vi "GetSetCtrls.vi"(8 "error in (no error)":errorcluster, 10 "Function (Load)":enum16{"Load", "Save"}(ring), 11 "Ini file (empty)":path) -> (0 "error out":errorcluster)   [LabVIEW 2011]
panel:
  out "Saved data":cluster{"Name":string, "Variant Data":variant}[](array[cluster])
  out "Initialized data":cluster{"Name":string, "Variant Data":variant}[](array[cluster])
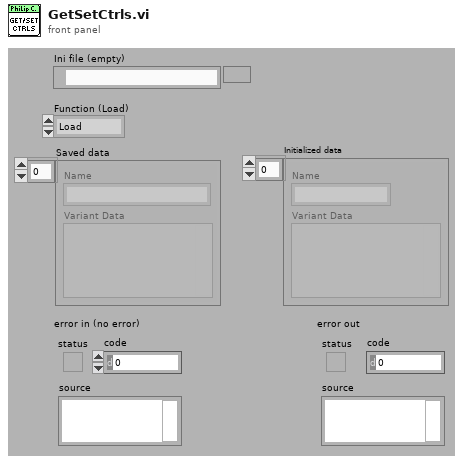
[diagram p1: front panel]
types:
  T1 = enum16{"open", "replace", "create", "open or create", "replace or create", "replace or create with confirmation"}
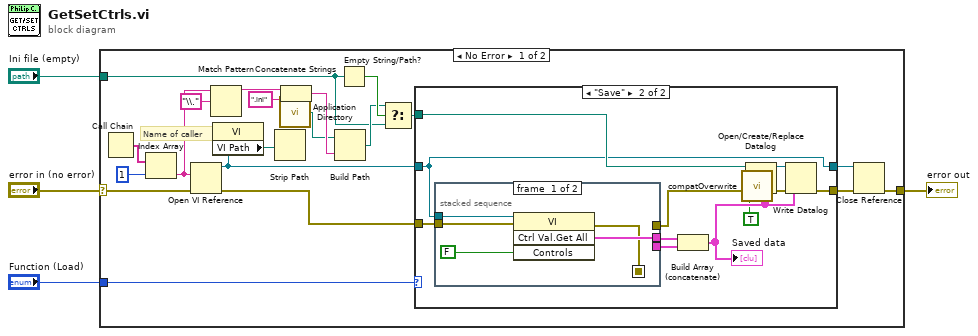
[diagram p0: block diagram]
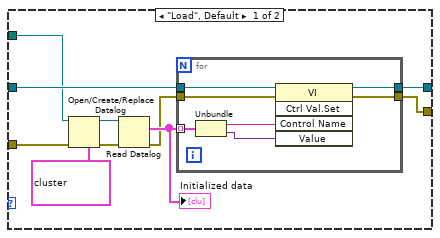
[diagram p2: hidden frame]
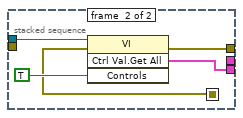
[diagram p3: hidden frame]
diagram:
  n1 = case shown="No Error" "error in (no error)" {
    selector: "error in (no error)" -> [w18 w64]
    tunnel: [w19 w64] -> w4
    tunnel: "Ini file (empty)" -> [w9 _]
    tunnel: "Function (Load)" -> [w8 _]
    frame No Error {
      # "Name of caller"
      n2 = Call Chain() -> (call chain=w24:string[])
      n3 = Index Array(array=w24, index=1) -> (element=w13:string)
      n4 = Open VI Reference(vi path=w13, error in (no error)=w18) -> (vi reference=w16:refnum<vi>, error out=w22:errorcluster)  [unwired: 4 in]
      n5 = Match Pattern(string=w13, regular expression="\\.") -> (before substring=w12:string)  [unwired: 1 in, 3 out]
      n6 = property class="VI"(reference=w16) -> ("VI Path"=w6:path)  [unwired: 1 in, 2 out]
      n7 = Strip Path(path=w6) -> ()  [unwired: 2 out]
      n8 = call <vilib>:"Application Directory.vi"() -> ("Application Directory"=w5:path)
      n9 = Concatenate Strings(w12, ".ini" ("Name of ini file 2")) -> (w11:string)
      n10 = Build Path(base path=w5, name or relative path=w11) -> (appended path=w10:path)
      n11 = Empty String/Path?(string/path=w9) -> (empty?=w17:bool)
      n12 = Select(t=w10, s=w17, f=w9) -> (s? t:f=w7:path)
      n13 = case shown="\"Save\"" w8 {
        tunnel: w7 -> [w25 w45]
        tunnel: w16 -> [w30 w43]
        tunnel: w22 -> [w28 w46]
        tunnel: [w27 w43] -> w21
        tunnel: [w26 w44] -> w20
        frame "Load", Default {
          n14 = Open/Create/Replace Datalog(5:cluster{"Name":string, "Variant Data":variant}[] [{"Name"="Numeric", "Variant Data"=variant(dbl 0.0)}, {"Name"="String", "Variant Data"=variant(string "")}, {"Name"="Controls", "Variant Data"=variant(bool TRUE)}] ("Get All Control Values [Variant] 2"), 8:w28, 11:w25) -> (0:w32:errorcluster, 3:w33:refnum<k1>)  [unwired: 3 in, 1 out]
          n15 = Read Datalog(4:w32, 7:w33) -> (0:w29:errorcluster, 2:w34:cluster{"Name":string, "Variant Data":variant}[])  [unwired: 1 in, 1 out]
          "Initialized data" <- w34
          n16 = for {
            tunnel: w34 -> [w41] mode=indexing
            tunnel: w30 -> [w38]
            tunnel: w29 -> [w37]
            tunnel: [w36] -> w26
            tunnel: [w35] -> w27
            n17 = Unbundle(w41) -> ("Name"=w40:string, "Variant Data"=w39:variant)
            n18 = invoke class="VI" method="Ctrl Val.Set"(reference=w38, error in=w37, "Control Name"=w40, "Value"=w39) -> (reference out=w35:refnum<vi>, error out=w36:errorcluster)  [unwired: 1 in, 3 out]
          }
        }
        frame "Save" {
          n19 = stacked-sequence {
            seq-local: [w54 _] -> [_ w59]
            tunnel: w43 -> [w58 w63]
            tunnel: [w57 _] -> w51
            tunnel: [_ w61] -> w52
            tunnel: [_ w60] -> w47
            tunnel: w46 -> [w55 _]
            frame #0 {
              n20 = invoke class="VI" method="Ctrl Val.Get All"(reference=w58, error in=w55, "Controls"=FALSE) -> (error out=w54:errorcluster, "Get All Control Values Variant"=w57:cluster{"Name":string, "Variant Data":variant}[])  [unwired: 1 in, 2 out]
            }
            frame #1 {
              n21 = invoke class="VI" method="Ctrl Val.Get All"(reference=w63, error in=w59, "Controls"=TRUE) -> (error out=w60:errorcluster, "Get All Control Values Variant"=w61:cluster{"Name":string, "Variant Data":variant}[])  [unwired: 1 in, 2 out]
            }
          }
          n22 = Build Array (concatenate)(w51, w52) -> (w53:cluster{"Name":string, "Variant Data":variant}[])
          "Saved data" <- w53
          n23 = call <vilib>:"compatOverwrite.vi"("overwrite (F)"=TRUE) -> ("overwrite?"=w42:T1)
          n24 = Open/Create/Replace Datalog(5:w53, 8:w47, 10:w42, 11:w45) -> (0:w48:errorcluster, 3:w49:refnum<k1>)  [unwired: 2 in, 1 out]
          n25 = Write Datalog(4:w48, 6:w53, 7:w49) -> (0:w44:errorcluster)  [unwired: 1 out]
        }
      }
      n26 = Close Reference(reference=w21, error in (no error)=w20) -> (error out=w19:errorcluster)
    }
    frame Error {
    }
  }
  "error out" <- w4
